vi "To Timestamp.vi"(8 "error in (no error)":errorcluster, 10 "milliseconds timer value":u32, 11 "Measurement Timer in":refnum<class "Measurement Timer.lvclass">) -> (0 "error out":errorcluster, 2 "Time Stamp Control":timestamp, 3 "Measurement Timer out":refnum<class "Measurement Timer.lvclass">)   [LabVIEW 2015, in "Measurement Timer.lvclass"]
uses:
  Measurement Timer.lvclass
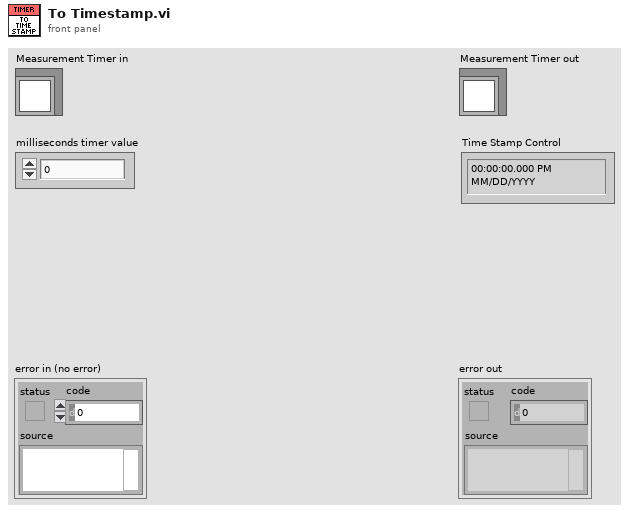
[diagram p1: front panel]
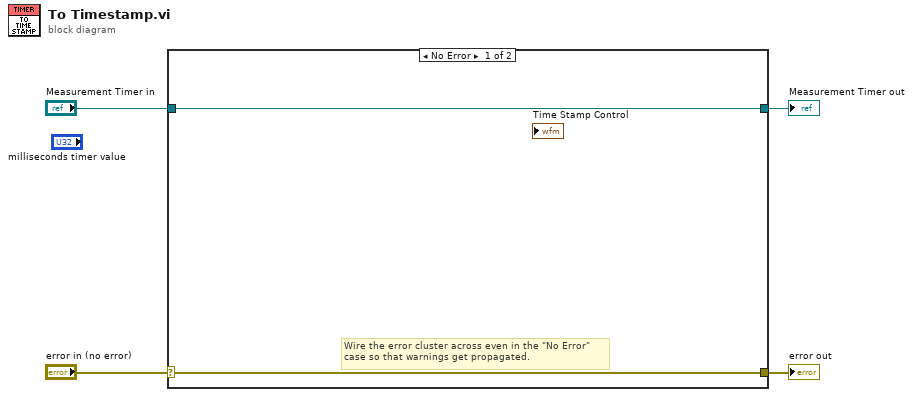
[diagram p0: block diagram]
diagram:
  n1 = case shown="No Error" "error in (no error)" {
    selector: "error in (no error)" -> [w5 w8]
    tunnel: [w5 w8] -> w3
    tunnel: [w6 w7] -> w1
    tunnel: "Measurement Timer in" -> [w6 w7]
    frame No Error {
      # "Wire the error cluster across even in the \"No Error\"\ncase so that warnings get propagated."
    }
    frame Error {
    }
  }
  "error out" <- w3
  "Measurement Timer out" <- w1
